vi "Stop Core.vi"(10 "final error code":i32, 11 "DAQ Actor in":refnum<class "DAQ Actor.lvclass">) -> (3 "DAQ Actor out":refnum<class "DAQ Actor.lvclass">)   [LabVIEW 2017, in "DAQ Actor.lvlib" / "DAQ Actor.lvclass"]
doc: "(<B>Filename</B>: Actor Framework.lvlib:Actor.lvclass:Stop Core.vi)\n\nDefines what the actor does before it stops. Use the <B>final error code</B> input to determine whether the actor shut down in response to an error.\n\nBy default, this method does nothing. A descendant class may override it to define behavior, such as shutting down any processes the actor initiated in its override of the Actor Core method."
uses:
  DAQ Actor.lvclass
  DAQ Actor.lvclass/DAQ Actor.ctl
  <vilib>/ActorFramework/Actor/Actor.lvclass
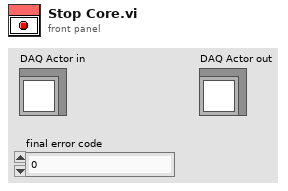
[diagram p1: front panel]
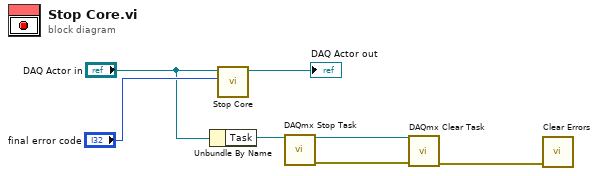
[diagram p0: block diagram]
diagram:
  n1 = Unbundle By Name("DAQ Actor in") -> ("Task"=w4:refnum<k21>)
  n2 = call-parent "Stop Core.vi"("final error code"="final error code", "Actor in"="DAQ Actor in") -> ("Actor out"=→"DAQ Actor out":refnum<class "DAQ Actor.lvclass">)  [unwired: 9 in]
  n3 = call <vilib>:"DAQmx Stop Task.vi"("task/channels in"=w4) -> ("task out"=w3:refnum<k21>, "error out"=w2:errorcluster)  [unwired: 13 in]
  n4 = call <vilib>:"DAQmx Clear Task.vi"("task in"=w3, "error in"=w2) -> ("error out"=w1:errorcluster)  [unwired: 13 in]
  n5 = call <vilib>:"Clear Errors.vi"("error in (no error)"=w1) -> ()  [unwired: 5 in, 2 out]
